vi "CRYGet Calibrated Device Name.vi"(0 "Calibration":T4 {"Calibration 2D"."Sens Curve"."Z data" items=["dB", "Lin"]; "Calibration 2D"."Sens Curve"."X data" items=["dB", "Lin"]; "Calibration 2D"."Sens Curve"."Y data" items=["dB", "Lin"]; "Calibration 2D"."Sens Curve"."Z dB ref" format="%.1f"; "Calibration 2D"."Sens Curve"."Z axis" items=["Log", "Lin"]; "Calibration 2D"."Sens Curve"."X dB ref" format="%.1f"; "Calibration 2D"."Sens Curve"."X axis" items=["Log", "Lin"]; "Calibration 2D"."Sens Curve"."Y axis" items=["Log", "Lin"]; "Calibration 2D"."Sens Curve"."Y dB ref" format="%.1f"; "Calibration 2D"."Sens Curve"."Curve"."z" format="%.2f"; "Calibration 2D"."Sens Curve"."Curve"."y" format="%.2f"; "Calibration 2D"."Sens Curve"."Curve"."x" format="%.2f"; "Calibration 2D"."EQ Curve"."Z data" items=["dB", "Lin"]; "Calibration 2D"."EQ Curve"."X data" items=["dB", "Lin"]; "Calibration 2D"."EQ Curve"."Y data" items=["dB", "Lin"]; "Calibration 2D"."EQ Curve"."Z dB ref" format="%.1f"; "Calibration 2D"."EQ Curve"."Z axis" items=["Log", "Lin"]; "Calibration 2D"."EQ Curve"."X dB ref" format="%.1f"; "Calibration 2D"."EQ Curve"."X axis" items=["Log", "Lin"]; "Calibration 2D"."EQ Curve"."Y axis" items=["Log", "Lin"]; "Calibration 2D"."EQ Curve"."Y dB ref" format="%.1f"; "Calibration 2D"."EQ Curve"."Curve"."z" format="%.2f"; "Calibration 2D"."EQ Curve"."Curve"."y" format="%.2f"; "Calibration 2D"."EQ Curve"."Curve"."x" format="%.2f"; "Calibration 2D"."Corr Curve"."Z data" items=["dB", "Lin"]; "Calibration 2D"."Corr Curve"."X data" items=["dB", "Lin"]; "Calibration 2D"."Corr Curve"."Y data" items=["dB", "Lin"]; "Calibration 2D"."Corr Curve"."Z dB ref" format="%.1f"; "Calibration 2D"."Corr Curve"."Z axis" items=["Log", "Lin"]; "Calibration 2D"."Corr Curve"."X dB ref" format="%.1f"; "Calibration 2D"."Corr Curve"."X axis" items=["Log", "Lin"]; "Calibration 2D"."Corr Curve"."Y axis" items=["Log", "Lin"]; "Calibration 2D"."Corr Curve"."Y dB ref" format="%.1f"; "Calibration 2D"."Corr Curve"."Curve"."z" format="%.2f"; "Calibration 2D"."Corr Curve"."Curve"."y" format="%.2f"; "Calibration 2D"."Corr Curve"."Curve"."x" format="%.2f"; "Calibration 2D"."Calibration"."EQ Step size" items=["R10", "R20", "R40", "R80", "User"]; "Calibration 2D"."Calibration"."Corr Step size" items=["R10", "R20", "R40", "R80", "User"]}) -> (1 "I_Signal Type Out":string[](array[string]), 2 "O_Signal Type Out":string[](array[string]), 3 "I_Calibration Out":T1[](array[typedef]) {"Sens Curve"."Z data" items=["dB", "Lin"]; "Sens Curve"."X data" items=["dB", "Lin"]; "Sens Curve"."Y data" items=["dB", "Lin"]; "Sens Curve"."Z dB ref" format="%.1f"; "Sens Curve"."Z axis" items=["Log", "Lin"]; "Sens Curve"."X dB ref" format="%.1f"; "Sens Curve"."X axis" items=["Log", "Lin"]; "Sens Curve"."Y axis" items=["Log", "Lin"]; "Sens Curve"."Y dB ref" format="%.1f"; "Sens Curve"."Curve"."z" format="%.2f"; "Sens Curve"."Curve"."y" format="%.2f"; "Sens Curve"."Curve"."x" format="%.2f"; "EQ Curve"."Z data" items=["dB", "Lin"]; "EQ Curve"."X data" items=["dB", "Lin"]; "EQ Curve"."Y data" items=["dB", "Lin"]; "EQ Curve"."Z dB ref" format="%.1f"; "EQ Curve"."Z axis" items=["Log", "Lin"]; "EQ Curve"."X dB ref" format="%.1f"; "EQ Curve"."X axis" items=["Log", "Lin"]; "EQ Curve"."Y axis" items=["Log", "Lin"]; "EQ Curve"."Y dB ref" format="%.1f"; "EQ Curve"."Curve"."z" format="%.2f"; "EQ Curve"."Curve"."y" format="%.2f"; "EQ Curve"."Curve"."x" format="%.2f"; "Corr Curve"."Z data" items=["dB", "Lin"]; "Corr Curve"."X data" items=["dB", "Lin"]; "Corr Curve"."Y data" items=["dB", "Lin"]; "Corr Curve"."Z dB ref" format="%.1f"; "Corr Curve"."Z axis" items=["Log", "Lin"]; "Corr Curve"."X dB ref" format="%.1f"; "Corr Curve"."X axis" items=["Log", "Lin"]; "Corr Curve"."Y axis" items=["Log", "Lin"]; "Corr Curve"."Y dB ref" format="%.1f"; "Corr Curve"."Curve"."z" format="%.2f"; "Corr Curve"."Curve"."y" format="%.2f"; "Corr Curve"."Curve"."x" format="%.2f"; "Calibration"."EQ Step size" items=["R10", "R20", "R40", "R80", "User"]; "Calibration"."Corr Step size" items=["R10", "R20", "R40", "R80", "User"]}, 4 "I_Name Out(Input Calibrated Name Out)":string[][](array[string]), 6 "O_Name Out(Output Calibrated Name Out)":string[][](array[string]), 10 "I_Calibrated Device Out":string[](array[string]), 14 "O_Calibration Out":T1[](array[typedef]) {"Sens Curve"."Z data" items=["dB", "Lin"]; "Sens Curve"."X data" items=["dB", "Lin"]; "Sens Curve"."Y data" items=["dB", "Lin"]; "Sens Curve"."Z dB ref" format="%.1f"; "Sens Curve"."Z axis" items=["Log", "Lin"]; "Sens Curve"."X dB ref" format="%.1f"; "Sens Curve"."X axis" items=["Log", "Lin"]; "Sens Curve"."Y axis" items=["Log", "Lin"]; "Sens Curve"."Y dB ref" format="%.1f"; "Sens Curve"."Curve"."z" format="%.2f"; "Sens Curve"."Curve"."y" format="%.2f"; "Sens Curve"."Curve"."x" format="%.2f"; "EQ Curve"."Z data" items=["dB", "Lin"]; "EQ Curve"."X data" items=["dB", "Lin"]; "EQ Curve"."Y data" items=["dB", "Lin"]; "EQ Curve"."Z dB ref" format="%.1f"; "EQ Curve"."Z axis" items=["Log", "Lin"]; "EQ Curve"."X dB ref" format="%.1f"; "EQ Curve"."X axis" items=["Log", "Lin"]; "EQ Curve"."Y axis" items=["Log", "Lin"]; "EQ Curve"."Y dB ref" format="%.1f"; "EQ Curve"."Curve"."z" format="%.2f"; "EQ Curve"."Curve"."y" format="%.2f"; "EQ Curve"."Curve"."x" format="%.2f"; "Corr Curve"."Z data" items=["dB", "Lin"]; "Corr Curve"."X data" items=["dB", "Lin"]; "Corr Curve"."Y data" items=["dB", "Lin"]; "Corr Curve"."Z dB ref" format="%.1f"; "Corr Curve"."Z axis" items=["Log", "Lin"]; "Corr Curve"."X dB ref" format="%.1f"; "Corr Curve"."X axis" items=["Log", "Lin"]; "Corr Curve"."Y axis" items=["Log", "Lin"]; "Corr Curve"."Y dB ref" format="%.1f"; "Corr Curve"."Curve"."z" format="%.2f"; "Corr Curve"."Curve"."y" format="%.2f"; "Corr Curve"."Curve"."x" format="%.2f"; "Calibration"."EQ Step size" items=["R10", "R20", "R40", "R80", "User"]; "Calibration"."Corr Step size" items=["R10", "R20", "R40", "R80", "User"]}, 15 "O_Calibrated Device Out":string[](array[string]))   [LabVIEW 2013]
uses:
  Typedef Control/CRYCalibration All Cluster.ctl
  Typedef Control/CRYCalibration 2DCluster.ctl
  Typedef Control/CRYCalibration Cluster.ctl
  Typedef Control/CRYData Cluster.ctl
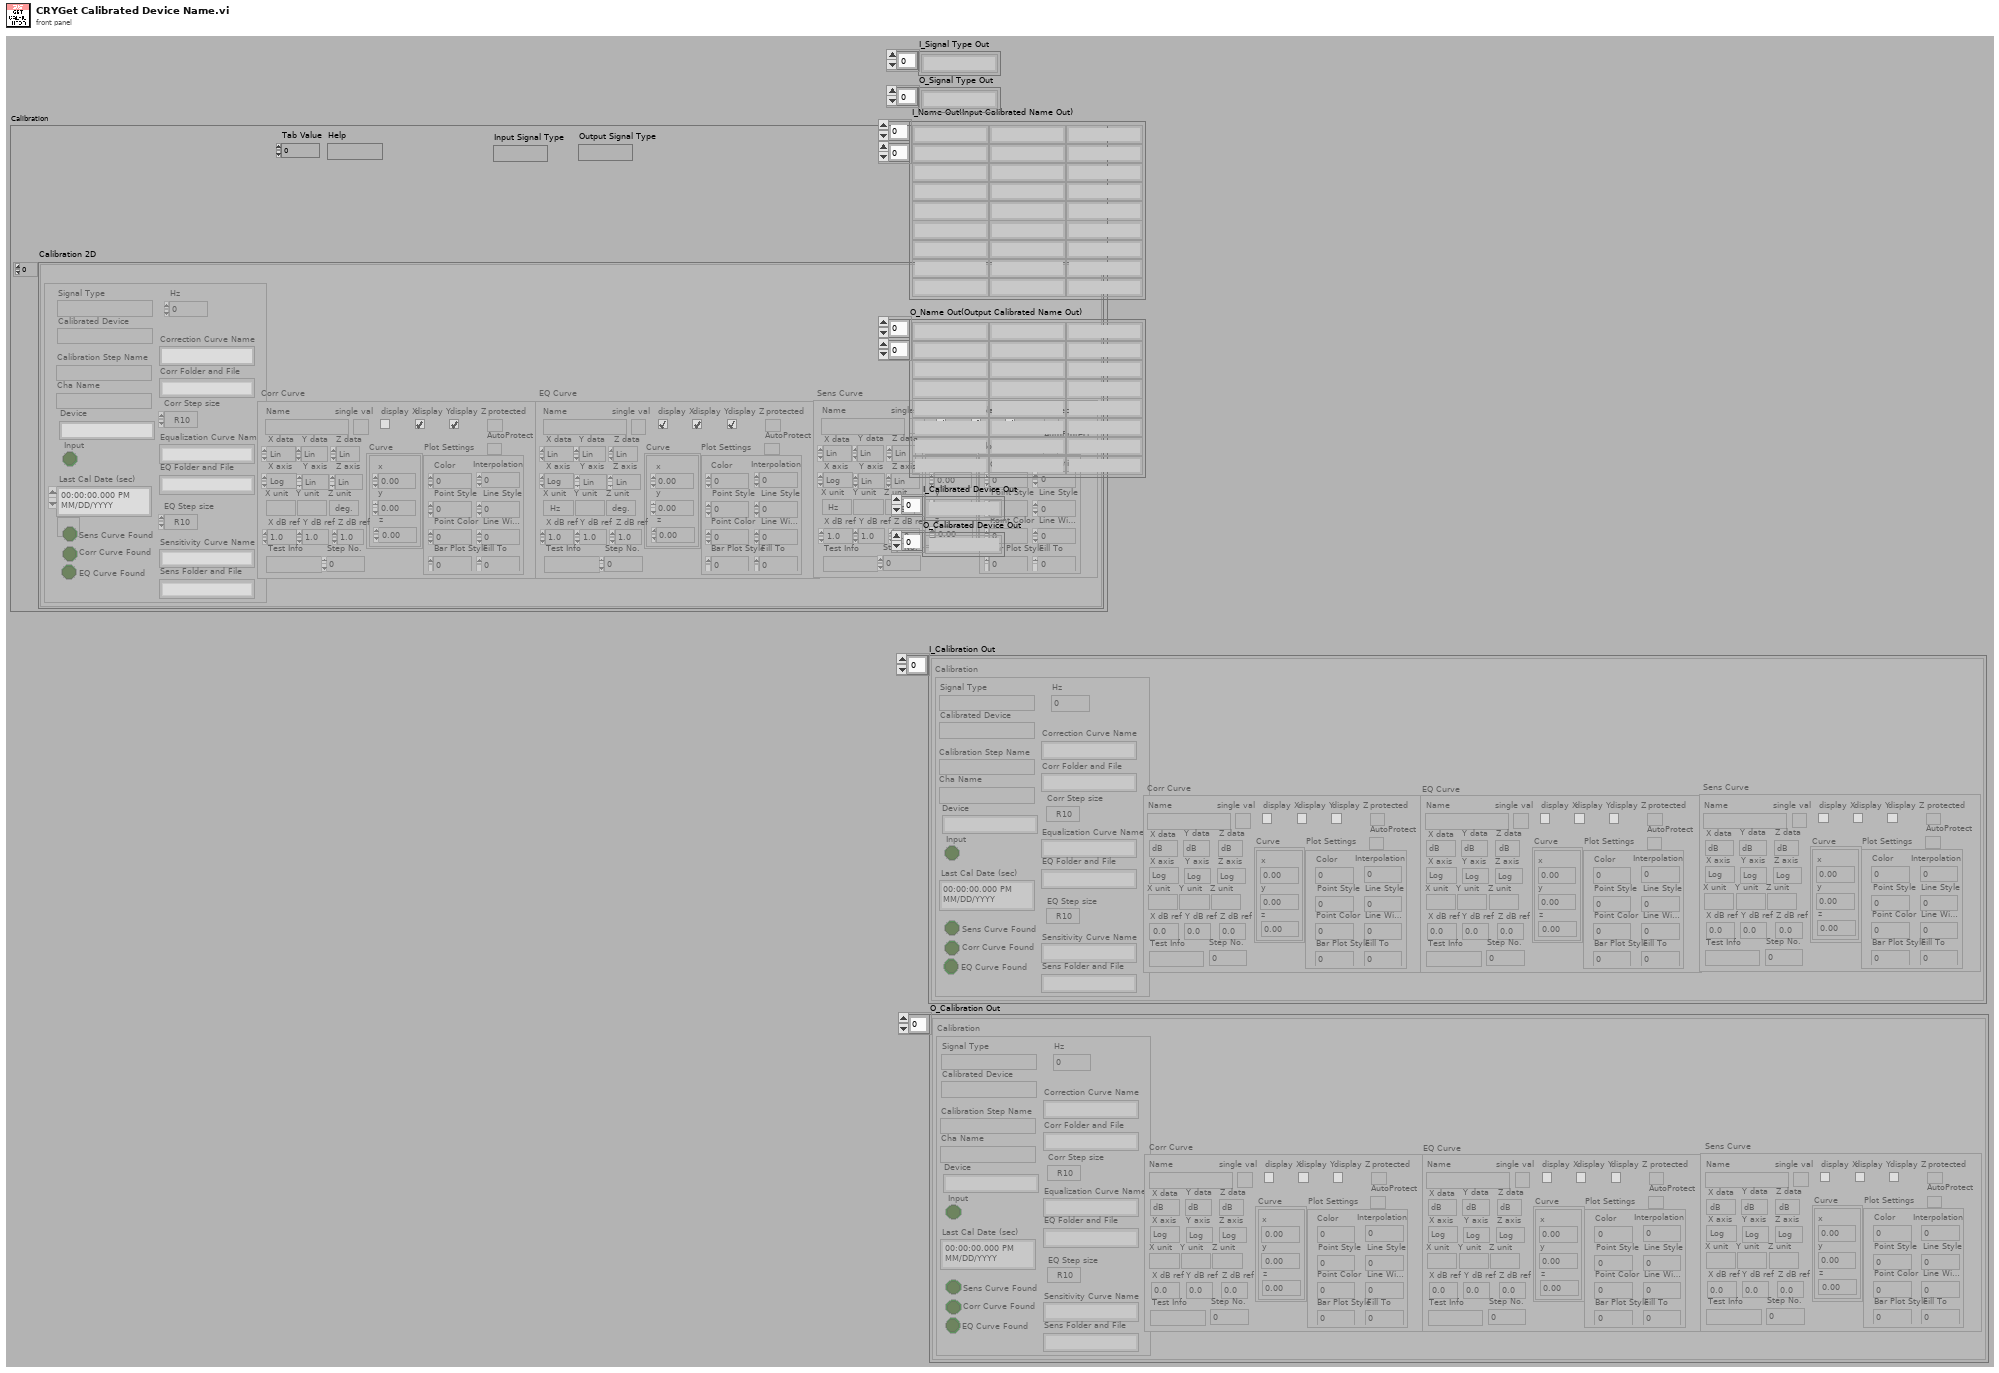
[diagram p1: front panel]
types:
  T1 = typedef "CRYCalibration 2DCluster.ctl" = cluster{"Calibration":T2, "Corr Curve":T3, "EQ Curve":T3, "Sens Curve":T3}
  T2 = typedef "CRYCalibration Cluster.ctl" = cluster{"Calibration Step Name":string, "Device":string, "Correction Curve Name":string, "Equalization Curve Name":string, "Sensitivity Curve Name":string, "Corr Folder and File":string, "EQ Folder and File":string, "Sens Folder and File":string, "Corr Step size":u16, "EQ Step size":u16, "Input":bool, "Last Cal Date (sec)":timestamp, "Cha Name":string, "Corr Curve Found":bool, "EQ Curve Found":bool, "Sens Curve Found":bool, "Signal Type":string, "Calibrated Device":string, "Hz":u32}
  T3 = typedef "CRYData Cluster.ctl" = cluster{"Name":string, "Curve":cluster{"x":dbl, "y":dbl, "z":dbl}[], "X data":u16, "Y data":u16, "Z data":u16, "X axis":u16, "Y axis":u16, "Z axis":u16, "X unit":string, "Y unit":string, "Z unit":string, "X dB ref":dbl, "Y dB ref":dbl, "Z dB ref":dbl, "single val":bool, "protected":bool, "display X":bool, "display Y":bool, "display Z":bool, "Test Info":string, "Step No.":i32, "Plot Settings":cluster{"Color":u32, "Interpolation":u8, "Point Style":u8, "Line Style":u8, "Point Color":u32, "Line Width":u8, "Bar Plot Style":u8, "Fill To":i16}, "AutoProtect":bool}
  T4 = typedef "CRYCalibration All Cluster.ctl" = cluster{"Calibration 2D":T1[], "Help":string, "Tab Value":i32, "Input Signal Type":string, "Output Signal Type":string}
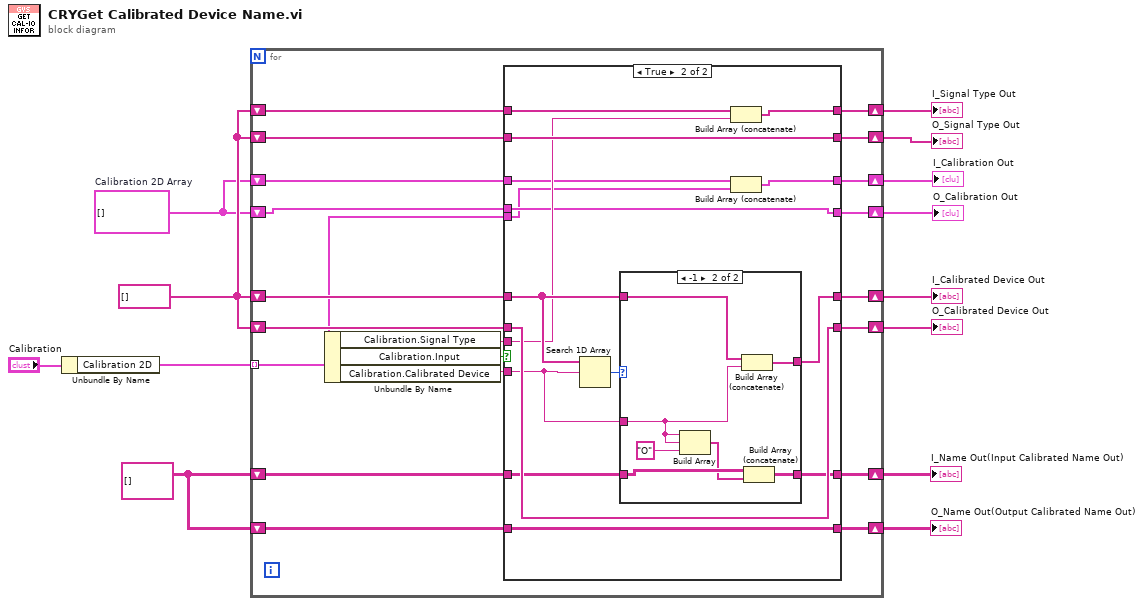
[diagram p0: block diagram]
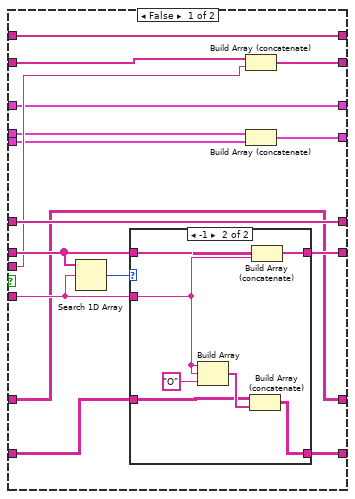
[diagram p2: hidden frame]
diagram:
  w2 = T1[] []  # Calibration 2D Array
  w11 = string[][] []
  w6 = string[] []
  n1 = Unbundle By Name("Calibration") -> ("Calibration 2D"=w12:T1[])
  n2 = for {
    tunnel: w12 -> [w18] mode=indexing
    shift-right: [w28] -> w8
    shift-left: w6 -> [w31]
    shift-right: [w29] -> w7
    shift-left: w6 -> [w30]
    shift-right: [w24] -> w9
    shift-left: w11 -> [w27]
    shift-right: [w25] -> w10
    shift-left: w11 -> [w26]
    shift-right: [w19] -> w5
    shift-left: w6 -> [w23]
    shift-right: [w21] -> w4
    shift-left: w6 -> [w22]
    shift-right: [w17] -> w3
    shift-left: w2 -> [w16]
    shift-right: [w14] -> w1
    shift-left: w2 -> [w15]
    n3 = Unbundle By Name(w18) -> ("Calibration.Signal Type"=w20:string, "Calibration.Input"=w32:bool, "Calibration.Calibrated Device"=w33:string)
    n4 = case shown="True" w32 {
      tunnel: w33 -> [w46 w73]
      tunnel: [w48 w71] -> w28
      tunnel: w31 -> [w48 w70]
      tunnel: w30 -> [w47 w74]
      tunnel: [w49 w74] -> w29
      tunnel: w27 -> [w42 w69]
      tunnel: [w44 w68] -> w25
      tunnel: w26 -> [w43 w68]
      tunnel: [w42 w67] -> w24
      tunnel: w23 -> [w41 w65]
      tunnel: w22 -> [w40 w66]
      tunnel: [w38 w66] -> w21
      tunnel: w20 -> [w39 w64]
      tunnel: [w41 w63] -> w19
      tunnel: w18 -> [w37 w59]
      tunnel: [w36 w60] -> w17
      tunnel: w16 -> [w35 w60]
      tunnel: w15 -> [w34 w62]
      tunnel: [w34 w61] -> w14
      frame False {
        n5 = Search 1D Array(1D array=w47, element=w46) -> (index of element=w45:i32)  [unwired: 1 in]
        n6 = case shown="-1" w45 {
          tunnel: [w51 w58] -> w49
          tunnel: w47 -> [w51 w57]
          tunnel: w46 -> [_ w55]
          tunnel: w43 -> [w50 w53]
          tunnel: [w50 w52] -> w44
          frame 0, Default {
          }
          frame -1 {
            n7 = Build Array(w55, w55, "O" ("Name")) -> (w54:string[])
            n8 = Build Array (concatenate)(w53, w54) -> (w52:string[][])
            n9 = Build Array (concatenate)(w57, w55) -> (w58:string[])
          }
        }
        n10 = Build Array (concatenate)(w40, w39) -> (w38:string[])
        n11 = Build Array (concatenate)(w35, w37) -> (w36:T1[])
      }
      frame True {
        n12 = Search 1D Array(1D array=w70, element=w73) -> (index of element=w72:i32)  [unwired: 1 in]
        n13 = case shown="-1" w72 {
          tunnel: [w76 w83] -> w71
          tunnel: w73 -> [_ w80]
          tunnel: w70 -> [w76 w81]
          tunnel: w69 -> [w75 w79]
          tunnel: [w75 w77] -> w67
          frame 0, Default {
          }
          frame -1 {
            n14 = Build Array(w80, w80, "O" ("Name")) -> (w78:string[])
            n15 = Build Array (concatenate)(w81, w80) -> (w83:string[])
            n16 = Build Array (concatenate)(w79, w78) -> (w77:string[][])
          }
        }
        n17 = Build Array (concatenate)(w65, w64) -> (w63:string[])
        n18 = Build Array (concatenate)(w62, w59) -> (w61:T1[])
      }
    }
  }
  "O_Name Out(Output Calibrated Name Out)" <- w10
  "I_Name Out(Input Calibrated Name Out)" <- w9
  "I_Calibrated Device Out" <- w8
  "O_Calibrated Device Out" <- w7
  "I_Signal Type Out" <- w5
  "O_Signal Type Out" <- w4
  "O_Calibration Out" <- w3
  "I_Calibration Out" <- w1
